vi "Export.vi"(8 "error in (no error)":errorcluster, 11 "Test Report in":refnum<class "Test Report.Template.lvclass">) -> (0 "error out":errorcluster, 3 "Test Report out":refnum<class "Test Report.Template.lvclass">)   [LabVIEW 2013, in "Caraya.lvlib" / "Test Report.Template.lvclass"]
uses:
  Test Report.Template.lvclass
  Test Report.Template.lvclass/Test Report.Template.ctl
  Test Report/Test Report.lvclass
  Test Result/Test Result.lvclass
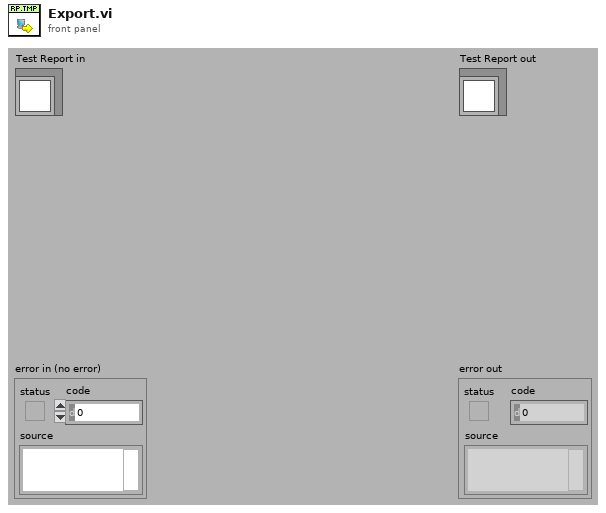
[diagram p1: front panel]
types:
  T1 = enum16{"open", "replace", "create", "open or create", "replace or create", "replace or create with confirmation"}
  T2 = typedef "Caraya.lvlib/Test Result.lvclass/Assert Event Data.ctl" = cluster{"Name":string, "Passed":bool, "Call Chain":string[], "Test Error":errorcluster, "Time Stamp":timestamp, "Unique Assert ID":string, "Test Key":string, "Execution time (s)":dbl, "Verbose Explanation":string}
  T3 = typedef "Caraya.lvlib/Test Result.lvclass/Test Node.ctl" = cluster{"Test Registration":T4, "Defined":bool, "Passed":bool}
  T4 = typedef "Caraya.lvlib/Test Result.lvclass/Test Registration Data.ctl" = cluster{"Name":string, "Call Chain":string[], "Time Stamp":timestamp}
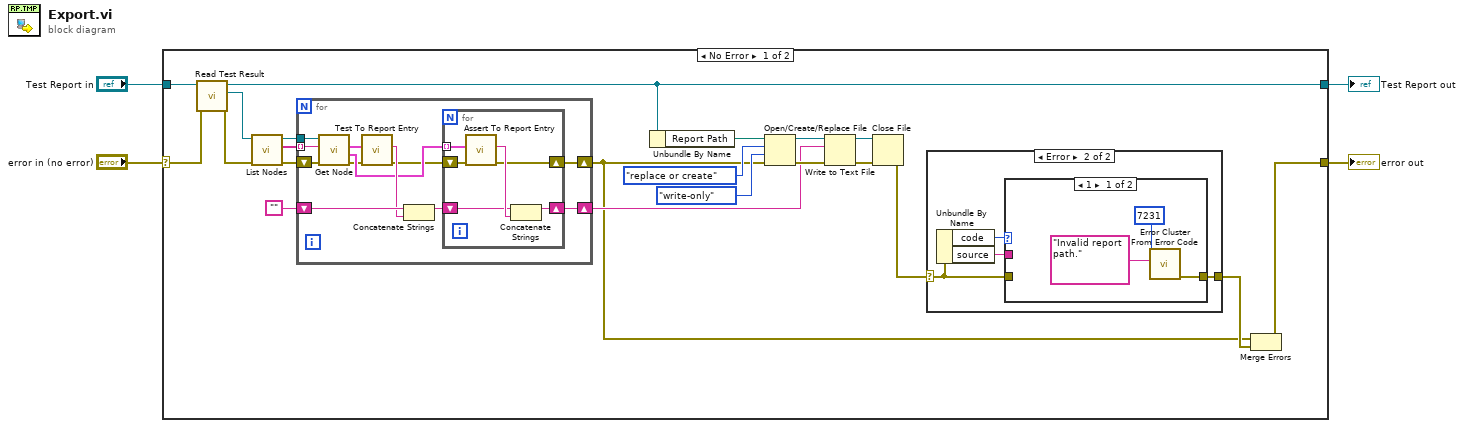
[diagram p0: block diagram]
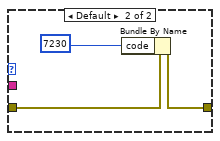
[diagram p3: hidden frame]
diagram:
  n1 = case shown="No Error" "error in (no error)" {
    selector: "error in (no error)" -> [w17 w56]
    tunnel: [w5 w56] -> w3
    tunnel: [w9 w55] -> w1
    tunnel: "Test Report in" -> [w18 w55]
    frame No Error {
      n2 = call "Read Test Result.vi"("error in (no error)"=w17, "Test Report in"=w18) -> ("error out"=w10:errorcluster, "Caraya.lvlib:Test Result.lvclass"=w16:refnum<class "Test Result.lvclass">, "Test Report out"=w9:refnum<class "Test Report.Template.lvclass">)  [unwired: 7 in]
      n3 = call "List Nodes.vi"("error in (no error)"=w10, "Test Result in"=w16) -> ("error out"=w11:errorcluster, "Nodes"=w15:string[], "Test Result out"=w14:refnum<class "Test Result.lvclass">)  [unwired: 7 in]
      n4 = for {
        tunnel: w15 -> [w47] mode=indexing
        tunnel: w14 -> [w48]
        shift-right: [w42] -> w12
        shift-left: "" -> [w45]
        shift-right: [w37] -> w6
        shift-left: w11 -> [w40]
        n5 = call "Get Node.vi"("error in (no error)"=w40, "Node"=w47, "Test Result in"=w48) -> ("error out"=w39:errorcluster, "Assertions"=w41:T2[], "Test Node"=w46:T3)  [unwired: 3 in, 3 out]
        n6 = call "Test To Report Entry.vi"("error in (no error)"=w39, "Test Node"=w46) -> ("error out"=w38:errorcluster, "String"=w44:string)  [unwired: 8 in]
        n7 = Concatenate Strings(w45, w44) -> (w43:string)
        n8 = for {
          shift-right: [w51] -> w42
          shift-left: w43 -> [w52]
          tunnel: w41 -> [w54] mode=indexing
          shift-right: [w49] -> w37
          shift-left: w38 -> [w50]
          n9 = call "Assert To Report Entry.vi"("error in (no error)"=w50, "Assert"=w54) -> ("error out"=w49:errorcluster, "String"=w53:string)  [unwired: 8 in]
          n10 = Concatenate Strings(w52, w53) -> (w51:string)
        }
      }
      n11 = Unbundle By Name(w9) -> ("Report Path"=w19:path)
      n12 = Open/Create/Replace File(file path (use dialog)=w19, error in=w6, operation (0:open)=T1."replace or create", access (0:read/write)=enum16{"read/write", "read-only", "write-only"}."write-only") -> (refnum out=w23:refnum<file>, error out=w22:errorcluster)  [unwired: 2 in, 1 out]
      n13 = Write to Text File(file (use dialog)=w23, text=w12, error in=w22) -> (refnum out=w21:refnum<file>, error out=w20:errorcluster)  [unwired: 1 in, 1 out]
      n14 = Close File(refnum=w21, error in=w20) -> (error out=w7:errorcluster)  [unwired: 1 out]
      n15 = case shown="Error" w7 {
        selector: w7 -> [w26 w29]
        tunnel: [w26 w30] -> w8
        frame No Error {
        }
        frame Error {
          n16 = Unbundle By Name(w29) -> ("code"=w28:i32, "source"=w27:string)
          n17 = case shown="1" w28 {
            tunnel: w29 -> [_ w36]
            tunnel: [w32 w35] -> w30
            tunnel: w27 -> [_ _]
            frame 1 {
              n18 = call <vilib>:"Error Cluster From Error Code.vi"("error message (\"\")"="Invalid report path." ("error message (\"\")"), "error code (0)"=7231) -> ("error out"=w32:errorcluster)  [unwired: 7 in]
            }
            frame Default {
              n19 = Bundle By Name(cluster=w36, "code"=7230 ("error code (0)")) -> (w35:errorcluster)
            }
          }
        }
      }
      n20 = Merge Errors(w6, w8) -> (w5:errorcluster)
    }
    frame Error {
    }
  }
  "error out" <- w3
  "Test Report out" <- w1
